vi "To Path Tree Data.vi"(10 "Path":path) -> (3 "Path Tree Data":refnum<class "Path.lvclass">)   [LabVIEW 2020, in "NI_VIAnCFGDataStructure.lvlib" / "Path.lvclass"]
doc: "Convert a Path value to Tree Data type."
uses:
  <vilib>/addons/analyzer/VIAnCFGDataStructure/Data Types/Path/Path.lvclass
  <vilib>/addons/analyzer/VIAnCFGDataStructure/Data Types/Path/Path.lvclass/Path.ctl
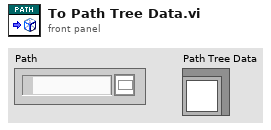
[diagram p1: front panel]
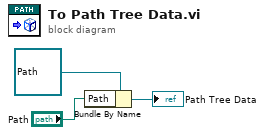
[diagram p0: block diagram]
diagram:
  n1 = Bundle By Name(cluster=refnum<class "Path.lvclass"> refnum ("Path in"), "Path"="Path") -> (→"Path Tree Data":refnum<class "Path.lvclass">)
